vi "R-Peak (SubVI).vi"(9 "detrend settings":T1, 10 "Denoised Signal":waveform(dbl), 11 "peaks/valleys":u16(ring) items=["peaks", "valleys"]) -> (1 "Amplitude":dbl[](array[numeric]), 2 "Location":dbl[](array[numeric]), 3 "Number of peaks":i32, 4 "Peak plot":cluster{"Ramp Pattern":dbl[], "X":dbl[]}[](graph))   [LabVIEW 2024]
uses:
  <vilib>/addons/Wavelet Analysis/application.llb/WA Multiscale Peak Detection (Waveform).vi
  <vilib>/addons/_Advanced Signal Processing/NI_AdvSigProcWA.lvlib
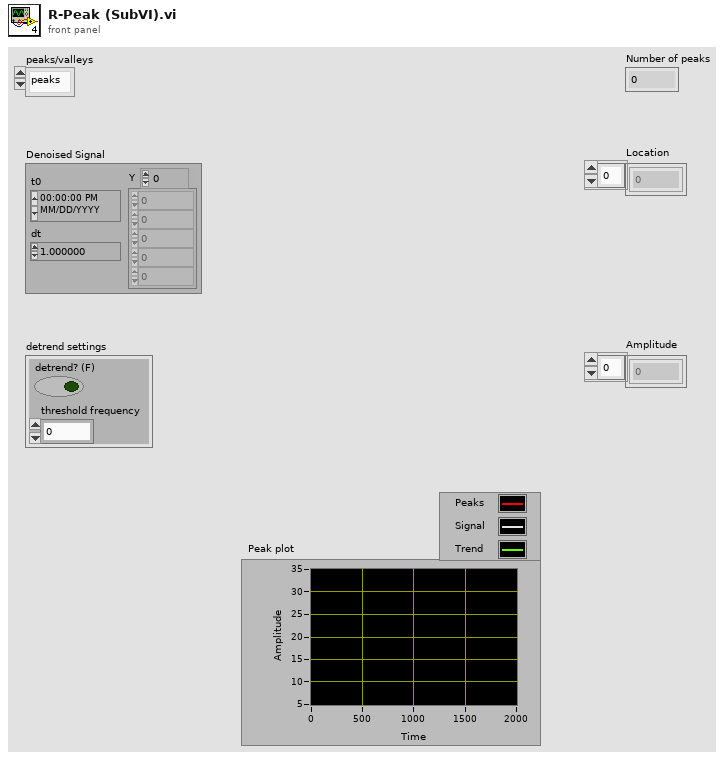
[diagram p1: front panel]
types:
  T1 = cluster{"detrend? (F)":bool, "threshold frequency":dbl}
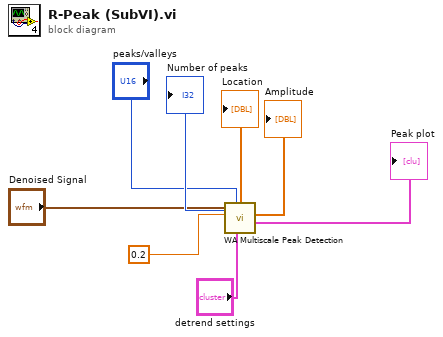
[diagram p0: block diagram]
diagram:
  n1 = call-poly <vilib>:"WA Multiscale Peak Detection.vi"("detrend settings"="detrend settings", "peaks/valleys"="peaks/valleys", "threshold"=0.2, "signal"="Denoised Signal") -> ("peak plot"=→"Peak plot":cluster{"Ramp Pattern":dbl[], "X":dbl[]}[], "amplitude"=→"Amplitude":dbl[], "location"=→"Location":dbl[], "number of peaks"=→"Number of peaks":i32)  [unwired: 3 in, 1 out]
